vi "ReadTDMSFileFromHBM&CorrectSpecial59.vi"(4 "error in (no error)":errorcluster, 6 "file path":path) -> (0 "sortie d'erreur":errorcluster, 2 "HBMWaveformsOut":waveform(dbl)[](graph))   [LabVIEW 2017]
panel:
  out "Graphe":waveform(dbl)[](graph)
  out "iteraFinal":i32
  out "TabNomFinal":string[](array[string])
  out "size(s) 2":i32
  out "Unit":string
  out "Name":string
  out "ChannelUnit":string[](array[string])
  out "ChannelNames":string[](array[string])
  out "Waveform Graph 2":waveform(dbl)(graph)
  out "WaveformHardware":waveform(dbl)[](graph)
  out "size(s)":i32
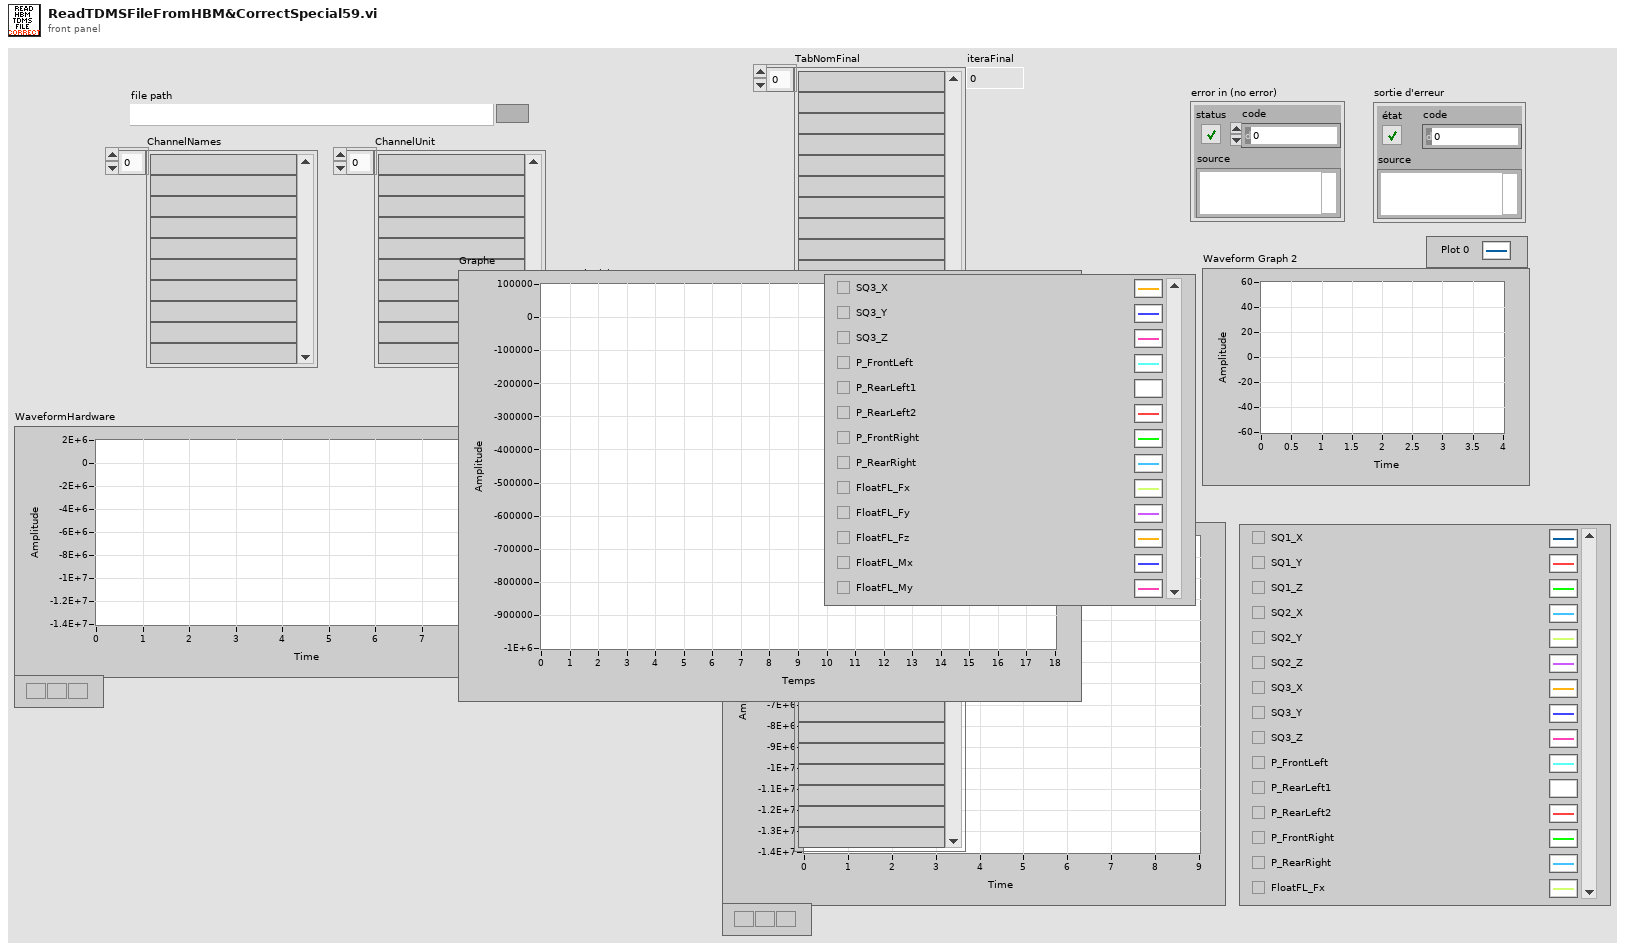
[diagram p1: front panel]
types:
  T1 = enum16{"open", "open or create", "create or replace", "create", "open (read-only)"}
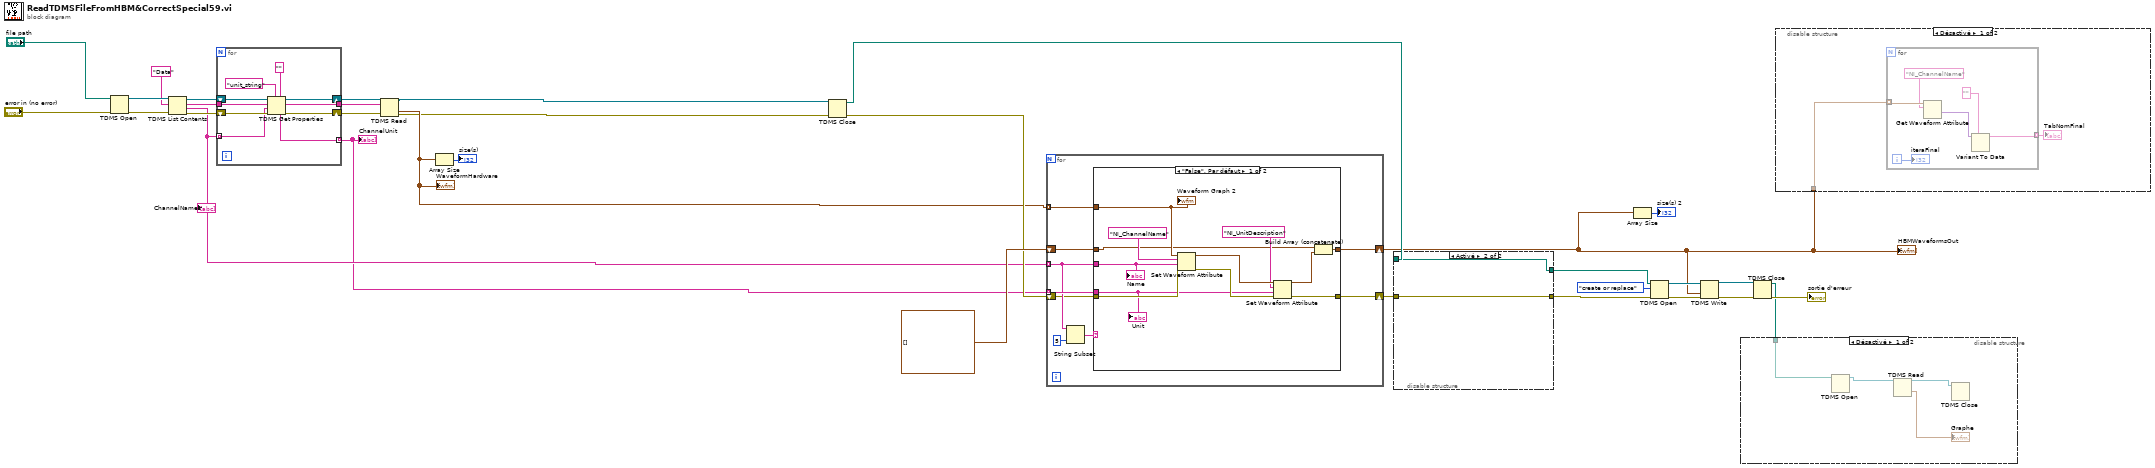
[diagram p0: block diagram]
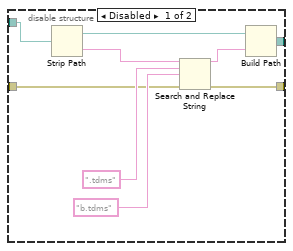
[diagram p2: hidden frame]
diagram:
  n1 = TDMS Open(8:"error in (no error)", 11:"file path") -> (0:w30:errorcluster, 3:w29:refnum<k34>)  [unwired: 5 in]
  n2 = TDMS List Contents(4:w30, 6:"Data" ("group name"), 7:w29) -> (0:w27:errorcluster, 1:w2:string[], 2:w25:string, 3:w28:refnum<k34>)
  "ChannelNames" <- w2
  n3 = for {
    tunnel: w25 -> [w38]
    shift-right: [w40] -> w24
    shift-left: w28 -> [w42]
    shift-right: [w39] -> w23
    shift-left: w27 -> [w41]
    tunnel: w2 -> [w35] mode=indexing
    tunnel: [w34] -> w1 mode=indexing
    tunnel: [w33] -> w22
    n4 = TDMS Get Properties(5:"" ("property name"), 7:"unit_string" ("property name"), 8:w41, 9:w35, 10:w38, 11:w42) -> (0:w39:errorcluster, 2:w33:string, 3:w40:refnum<k34>, 4:w34:string)  [unwired: 2 out]
  }
  "ChannelUnit" <- w1
  n5 = TDMS Read(0:w24, 5:w22, 11:w23) -> (4:w4:refnum<k34>, 10:w5:waveform(dbl)[], 15:w3:errorcluster)  [unwired: 5 in, 3 out]
  "WaveformHardware" <- w5
  n6 = Array Size(array=w5) -> (size(s)=→"size(s)":i32)
  n7 = TDMS Close(8:w3, 11:w4) -> (0:w19:errorcluster, 3:w9:path)
  n8 = for {
    tunnel: w5 -> [w51] mode=indexing
    tunnel: w2 -> [w48] mode=indexing
    tunnel: w1 -> [w50] mode=indexing
    shift-right: [w45] -> w7
    shift-left: waveform(dbl)[] [] -> [w44]
    shift-right: [w49] -> w11
    shift-left: w19 -> [w43]
    n9 = String Subset(string=w48, length (rest)=5 ("length (rest)")) -> (substring=w46:string)  [unwired: 1 in]
    n10 = case shown="\"False\", Par défaut" w46 {
      tunnel: w43 -> [w63 w64]
      tunnel: w51 -> [w62 _]
      tunnel: w50 -> [w57 _]
      tunnel: [w56 w64] -> w49
      tunnel: w48 -> [w55 _]
      tunnel: [w53 w65] -> w45
      tunnel: w44 -> [w52 w65]
      frame "False", Default {
        n11 = Set Waveform Attribute(4:w63, 5:w55, 6:"NI_ChannelName" ("name"), 7:w62) -> (0:w61:errorcluster, 3:w60:waveform(dbl))  [unwired: 1 out]
        n12 = Set Waveform Attribute(4:w61, 5:w57, 6:"NI_UnitDescription" ("name"), 7:w60) -> (0:w56:errorcluster, 3:w54:waveform(dbl))  [unwired: 1 out]
        n13 = Build Array (concatenate)(w52, w54) -> (w53:waveform(dbl)[])
        "Waveform Graph 2" <- w62
        "Name" <- w55
        "Unit" <- w57
      }
      frame "Temps" {
      }
    }
  }
  "HBMWaveformsOut" <- w7
  n14 = disable-structure shown="Activé" {
    disable-tunnel: w11 -> [w72 w75]
    disable-tunnel: [w71 w75] -> w10
    disable-tunnel: w9 -> [w70 w76]
    disable-tunnel: [w66 w76] -> w8
    frame Disabled {
      n15 = Strip Path(path=w70) -> (stripped path=w68:path, name=w69:string)
      n16 = Search and Replace String(input string=w69, search string=".tdms" ("sous-chaîne (\"\")"), replace string="b.tdms" ("sous-chaîne (\"\")"), error in=w72) -> (result string=w67:string, error out=w71:errorcluster)  [unwired: 4 in, 2 out]
      n17 = Build Path(base path=w68, name or relative path=w67) -> (appended path=w66:path)
    }
    frame Enabled {
    }
  }
  n18 = Array Size(array=w7) -> (size(s)=→"size(s) 2":i32)
  n19 = TDMS Open(8:w10, 10:T1."create or replace" ("opération (0 : open)"), 11:w8) -> (0:w18:errorcluster, 3:w16:refnum<k34>)  [unwired: 4 in]
  n20 = TDMS Write(0:w16, 9:w7, 11:w18) -> (4:w15:refnum<k34>, 15:w17:errorcluster)  [unwired: 3 in, 2 out]
  n21 = TDMS Close(8:w17, 11:w15) -> (0:→"sortie d'erreur":errorcluster, 3:w6:path)
  n22 = disable-structure shown="Désactivé" {
    disable-tunnel: w6 -> [w80 _]
    frame Disabled {
      n23 = TDMS Open(11:w80) -> (3:w79:refnum<k34>)  [unwired: 6 in, 1 out]
      n24 = TDMS Read(0:w79) -> (4:w78:refnum<k34>, 10:→"Graphe":waveform(dbl)[])  [unwired: 7 in, 4 out]
      n25 = TDMS Close(11:w78) -> ()  [unwired: 1 in, 2 out]
    }
    frame Enabled {
    }
  }
  n26 = disable-structure shown="Désactivé" {
    disable-tunnel: w7 -> [w82 _]
    frame Disabled {
      n27 = for {
        tunnel: w82 -> [w88] mode=indexing
        tunnel: [w84] -> w81 mode=indexing
        i -> [w83]
        n28 = Get Waveform Attribute(6:"NI_ChannelName" ("name"), 7:w88) -> (1:w86:variant)  [unwired: 2 in, 3 out]
        n29 = Variant To Data(type="" ("name"), Variant=w86) -> (data=w84:string)  [unwired: 1 in, 1 out]
        "iteraFinal" <- w83
      }
      "TabNomFinal" <- w81
    }
    frame Enabled {
    }
  }
